vi "clipconf.vi"() -> ()   [LabVIEW 2009]
uses:
  <vilib>/Utility/NIReport.llb/NI_report.lvclass
  <instrlib>/Agilent 81150/Agilent 81150.lvlib
  <vilib>/Analysis/NI_AALBase.lvlib
panel:
  out "Instrument VISA out":T1
  in  "conf value":i32[](array[numeric])=[200, 220, 250, 180, 150, 120, 100, 300]
  in  "Fotoelecton to clip":i32[](array[numeric])=[0, 12, 11, 10, 9, 8, 7, 6]
  out "Numeric 3":i32
  out "error out":errorcluster
  out "Quantity bucle":i32=62
  out "mean value":dbl=711.9915188935893
  in  "Voltages comprobation":dbl[](array[numeric])=[0.05, 0.1, 0.2, 0.3, 0.35, 0.4, 0.45, 0.5, 0.55, 0.6, 0.7, 0.8, 0.9, 1.0, 1.2, 1.5, 1.8, 2.0]
  out "L1 values":i32[](array[numeric])=[75, 76, 78, 63, 67, 69]
  out "L1 values":i32[](array[numeric])=[350, 351, 357, 318, 319, 317]
  out "Vatt":i32[](array[numeric])=[2200, 2200, 2200, 2200, 2200, 2200]
  out "Vclip":i32[](array[numeric])=[415, 417, 409, 455, 424, 466]
  in  "Vatt ini":i32[](array[numeric])=[1500, 1500, 1500, 1500, 1500, 1500, 1500]
  in  "Vclip ini":i32[](array[numeric])=[0, 0, 0, 0, 0, 0, 0]
  in  "Comprobation":bool=TRUE
  in  "Channels":i32[](array[numeric])=[0, 1, 2, 3, 4, 5, 6]
  in  "Cycles Burst":i32=10000
  out "IPR_Address":i32=23
  out "L1 Address":i32=17
  in  "L1 version":bool
  in  "Instrument VISA in":T1={"AWG VISA"="81160A", "Oscilloscope  VISA "="DSO80204B", "Integration Board IP"="172.16.7.43", "connection ID"=refnum, "report out"=refnum, "report file path"=path "D:/CTA/Data_test"}
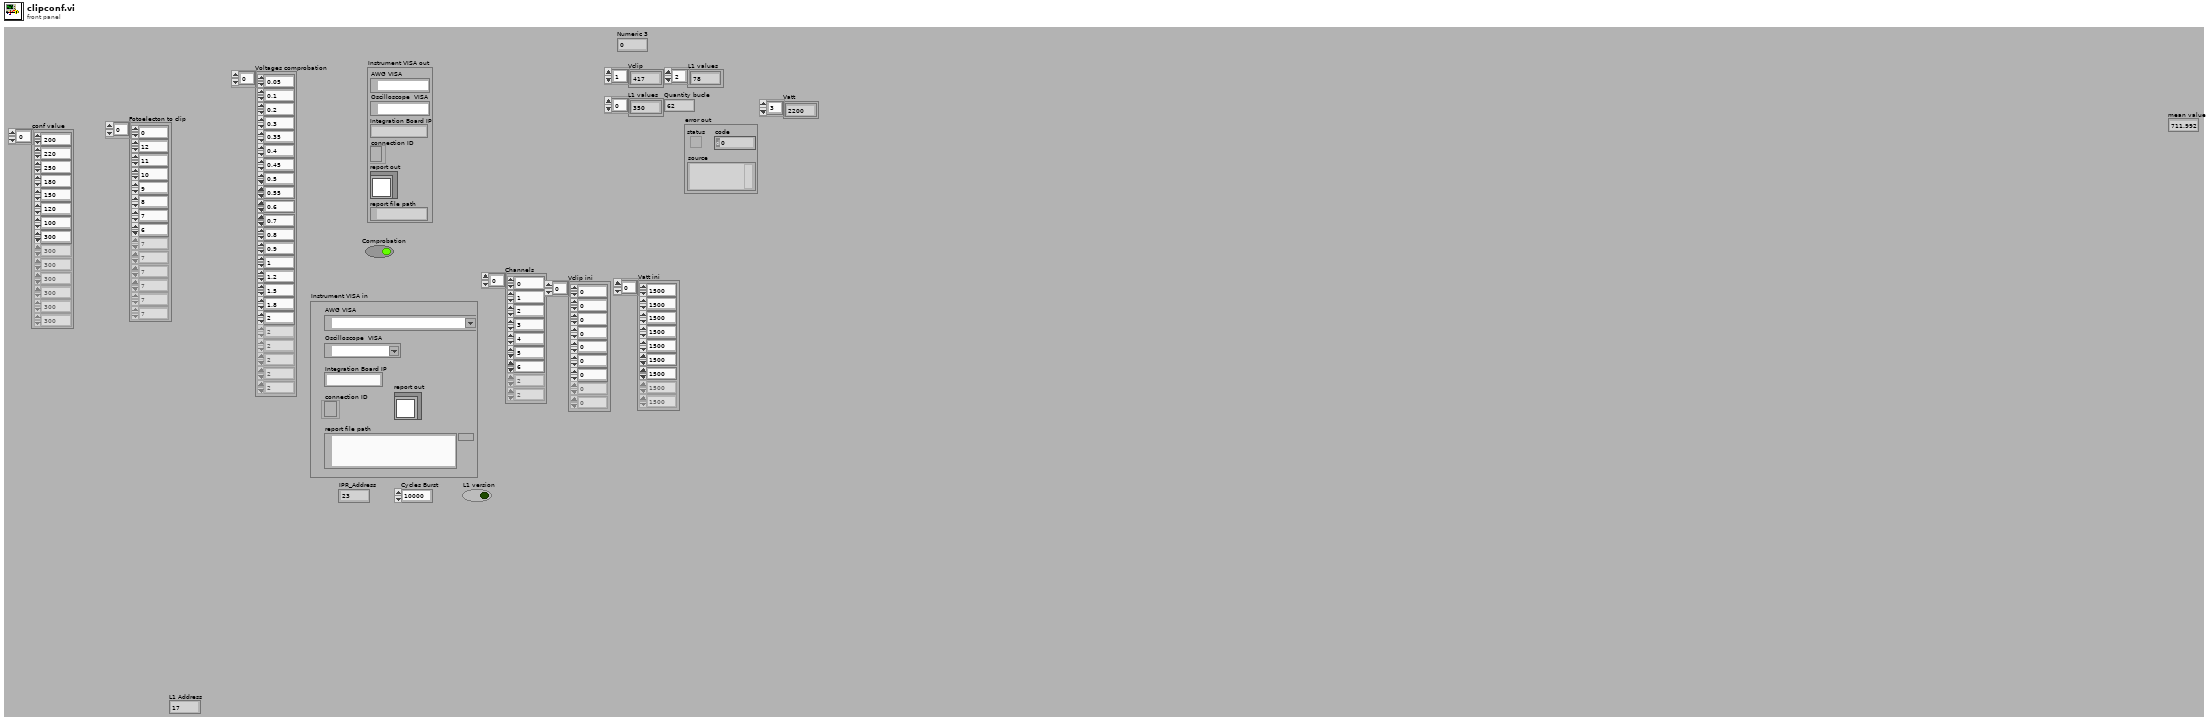
[diagram p1: front panel]
types:
  T1 = cluster{"AWG VISA":refnum<visa-resource-name>, "Oscilloscope  VISA ":refnum<visa-resource-name>, "Integration Board IP":string, "connection ID":refnum<k5>, "report out":refnum<class "NI_report.lvclass">, "report file path":path}
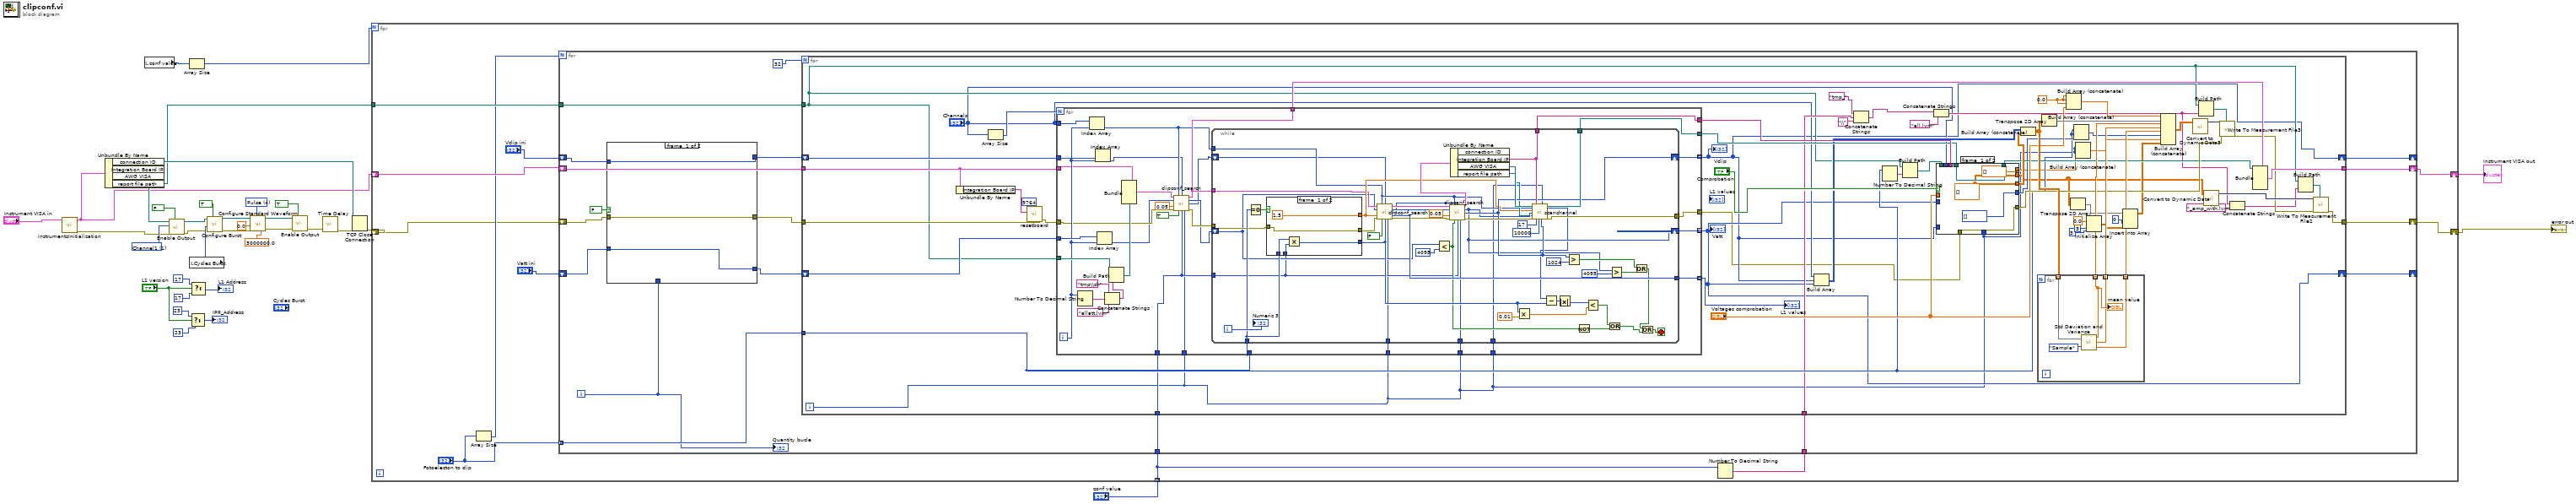
[diagram p0: block diagram]
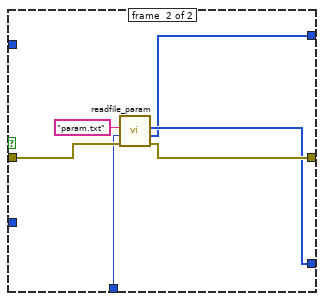
[diagram p2: hidden frame]
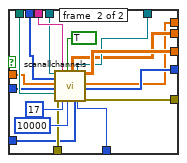
[diagram p3: hidden frame]
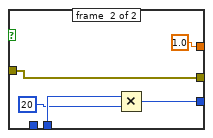
[diagram p4: hidden frame]
diagram:
  w26 = u16 4 items=["Sine", "Square", "Ramp Up", "Ramp Down", "Pulse", "Noise", "DC"] ("Waveform (0: Sine)")
  w32 = u16 1 items=["Channel1"=1, "Channel2"=2] ("Channel (1: Channel1)")
  n1 = call "instrumentsInitialization.vi"("Instrument VISA in"="Instrument VISA in") -> ("error out"=w11:errorcluster, "Instrument VISA out"=w1:T1)  [unwired: 9 in]
  n2 = Unbundle By Name(w1) -> ("connection ID"=w14:refnum<k5>, "AWG VISA"=w27:refnum<visa-resource-name>, "report file path"=w7:path)  [unwired: 1 out]
  n3 = local read "conf value"() -> (w35:i32[])
  n4 = call <instrlib>:"Enable Output.vi"("Enable Output (T: Enable)"=FALSE, "error in (no error)"=w11, "Channel (1: Channel1)"=w32, "VISA resource name"=w27) -> ("error out"=w13:errorcluster, "VISA resource name out"=w12:refnum<visa-resource-name>)  [unwired: 6 in]
  n5 = Array Size(array=w35) -> (size(s)=w5:i32)
  n6 = local read "Cycles Burst"() -> (w15:i32)
  n7 = Select(t=23 ("Address"), s="L1 version", f=23 ("Address")) -> (s? t:f=→"IPR_Address":i32)
  n8 = Select(t=17 ("Address"), s="L1 version", f=17 ("Address")) -> (s? t:f=→"L1 Address":i32)
  n9 = call <instrlib>:"Configure Burst.vi"("Enable Burst (F: Disable)"=TRUE, "error in (no error)"=w13, "Burst Count (2)"=w15, "VISA resource name"=w12) -> ("error out"=w23:errorcluster, "VISA resource name out"=w24:refnum<visa-resource-name>)  [unwired: 6 in]
  n10 = call <instrlib>:"Configure Standard Waveform.vi"("Frequency (1000.0 Hz)"=3000000.0, "Waveform (0: Sine)"=w26, "error in (no error)"=w23, "Amplitude (1.0 Vpp)"=0.0, "VISA resource name"=w24) -> ("error out"=w22:errorcluster, "VISA resource name out"=w10:refnum<visa-resource-name>)  [unwired: 5 in]
  n11 = call <instrlib>:"Enable Output.vi"("Enable Output (T: Enable)"=TRUE, "error in (no error)"=w22, "VISA resource name"=w10) -> ("error out"=w8:errorcluster)  [unwired: 7 in, 1 out]
  n12 = call "Time Delay"("error in (no error)"=w8) -> ("error out"=w9:errorcluster)  [unwired: 10 in]
  n13 = TCP Close Connection(connection ID=w14, error in (no error)=w9) -> (error out=w2:errorcluster)  [unwired: 1 in, 1 out]
  n14 = for {
    N: w5 -> [_]
    tunnel: w7 -> [w46]
    tunnel: "conf value" -> [w44] mode=indexing
    shift-right: [w43] -> w3
    shift-left: w1 -> [w42]
    shift-right: [w45] -> w6
    shift-left: w2 -> [w36]
    n15 = Array Size(array="Fotoelecton to clip") -> (size(s)=w40:i32)
    n16 = Number To Decimal String(number=w44) -> (decimal integer string=w39:string)  [unwired: 1 in]
    n17 = for {
      N: w40 -> [_]
      tunnel: w46 -> [w58]
      shift-right: [w56] -> _
      shift-left: "Vatt ini" -> [w52]
      shift-right: [w55] -> _
      shift-left: "Vclip ini" -> [w53]
      shift-right: [w64] -> w43
      shift-left: w42 -> [w63]
      shift-right: [w59] -> w45
      shift-left: w36 -> [w50]
      tunnel: "Fotoelecton to clip" -> [w62] mode=indexing
      tunnel: w44 -> [w61]
      tunnel: w39 -> [w60]
      i -> [w48]
      n18 = case shown="False" FALSE {
        tunnel: w50 -> [w67 w73]
        tunnel: [w67 w72] -> w49
        tunnel: [w65 w71] -> w51
        tunnel: [w66 w70] -> w54
        tunnel: w53 -> [w66 _]
        tunnel: w52 -> [w65 _]
        tunnel: w48 -> [_ w69]
        frame #0 {
        }
        frame #1 {
          n19 = call "readfile_param.vi"("error in"=w73, "index"=w69, "file"="param.txt") -> ("error out"=w72:errorcluster, "clipping"=w70:i32[], "attenuation"=w71:i32[])  [unwired: 4 in, 1 out]
        }
      }
      n20 = for {
        N: 32 -> [_]
        tunnel: [w123] -> w64
        tunnel: w49 -> [w111]
        tunnel: w63 -> [w109]
        tunnel: w62 -> [w103]
        tunnel: w61 -> [w102]
        tunnel: w60 -> [w98]
        tunnel: [w95] -> w59
        tunnel: w58 -> [w93]
        shift-right: [w77] -> w56
        shift-left: w51 -> [w135]
        shift-right: [w76] -> w55
        shift-left: w54 -> [w106]
        i -> [w75]
        w114 = 0.0 ("element")
        n21 = Unbundle By Name(w109) -> ("Integration Board IP"=w108:string)
        n22 = Array Size(array="Channels") -> (size(s)=w79:i32)
        n23 = call "resetboard.vi"("error in (no error)"=w111, "address"=w108, "remote port or service name"=u16 9764) -> ("error out"=w110:errorcluster)  [unwired: 7 in, 1 out]
        n24 = for {
          N: w79 -> [_]
          tunnel: w106 -> [w196]
          tunnel: "Channels" -> [w194]
          tunnel: w109 -> [w185]
          tunnel: w135 -> [w195]
          tunnel: [w189] -> w133
          tunnel: w93 -> [w198]
          tunnel: [w187] -> w77 mode=indexing
          tunnel: w110 -> [w178]
          tunnel: [w190] -> w74
          tunnel: [w183] -> w76 mode=indexing
          tunnel: [w188] -> w131 mode=indexing
          tunnel: [w182] -> w122
          tunnel: [w180] -> w124
          tunnel: w103 -> [w181]
          tunnel: w102 -> [w169]
          tunnel: w75 -> [w168]
          tunnel: w75 -> [w167]
          tunnel: w75 -> [w166]
          tunnel: w75 -> [w165]
          i -> [w186]
          n25 = Number To Decimal String(number=w186) -> (decimal integer string=w197:string)  [unwired: 1 in]
          n26 = Index Array(array=w194, index=w186) -> (element=w174:i32)
          n27 = Index Array(array=w196, index=w186) -> (element=w173:i32)
          n28 = Index Array(array=w195, index=w186) -> (element=w176:i32)
          n29 = Concatenate Strings("tmp\\ch" ("name or relative path"), w197, "allatt.lvm" ("string")) -> (w193:string)
          n30 = Build Path(base path=w198, name or relative path=w193) -> (appended path=w184:path)
          n31 = Bundle(cluster=w185, "report file path"=w184) -> (w179:T1)  [unwired: 5 in]
          n32 = call "clipconf_search.vi"("input cluster"=w179, "Channel"=w174, "vclip"=w173, "Vatt init"=w176, "Voltage value"=0.05, "error out 2"=w178, "Att/clip"=TRUE, "conf value"=w169, "Delay"=w168) -> ("output cluster"=w180:T1, "Vatt init"=w175:i32, "vclip"=w172:i32, "error out"=w177:errorcluster)  [unwired: 2 in, 1 out]
          n33 = while {
            tunnel: w177 -> [w208]
            tunnel: [w231] -> w190
            tunnel: [w234] -> w189
            tunnel: w174 -> [w206]
            shift-right: [w228] -> w183
            shift-left: w172 -> [w204]
            tunnel: [w247] -> w188
            shift-right: [w227] -> w187
            shift-left: w175 -> [w203]
            tunnel: w180 -> [w205]
            tunnel: [w233] -> w182
            tunnel: w181 -> [w212]
            tunnel: w169 -> [w202]
            tunnel: w167 -> [w201]
            tunnel: w166 -> [w200]
            tunnel: w165 -> [w199]
            i -> [w218]
            stop <- w246 stop-if-true
            n34 = Equal To 0?(x=w212) -> (x = 0?=w219:bool)
            n35 = case shown="False" w219 {
              tunnel: [1.5 ("Voltage value") 1.0 ("Voltage value")] -> w220
              tunnel: w202 -> [w250 w257]
              tunnel: [w251 w254] -> w213
              tunnel: w212 -> [w249 _]
              tunnel: w208 -> [w248 w253]
              tunnel: [w248 w253] -> w207
              frame #0 {
                n36 = Multiply(x=w249, y=w250) -> (x*y=w251:i32)
              }
              frame #1 {
                n37 = Multiply(x=w257, y=20) -> (x*y=w254:i32)
              }
            }
            n38 = call "clipconf_search.vi"("input cluster"=w205, "Channel"=w206, "vclip"=w204, "Vatt init"=w203, "Voltage value"=w220, "error out 2"=w207, "Att/clip"=FALSE, "conf value"=w213, "Delay"=w201) -> ("output cluster"=w241:T1, "Vatt init"=w239:i32, "vclip"=w211:i32, "L1 value"=w247:i32, "error out"=w242:errorcluster)  [unwired: 2 in]
            n39 = Less?(x=w203, y=4095) -> (x < y?=w210:bool)
            n40 = call "clipconf_search.vi"("input cluster"=w241, "Channel"=w206, "vclip"=w211, "Vatt init"=w239, "Voltage value"=0.05, "error out 2"=w242, "Att/clip"=w210, "conf value"=w202, "Delay"=w200) -> ("output cluster"=w240:T1, "Vatt init"=w227:i32, "vclip"=w228:i32, "error out"=w232:errorcluster)  [unwired: 2 in, 1 out]
            n41 = Unbundle By Name(w240) -> ("Integration Board IP"=w234:string, "AWG VISA"=w235:refnum<visa-resource-name>, "report file path"=w226:path)  [unwired: 1 out]
            n42 = Multiply(x=w213, y=0.01) -> (x*y=w221:dbl)
            n43 = call "scanchannel.vi"("VISA resource name out"=w235, "num ch"=w206, "Voltage value"=w220, "Init vatt value"=w227, "base path"=w226, "error in"=w232, "Integration Board IP"=w234, "L1 Address"=17, "Ch burst"=10000, "Delay"=w199, "vclip"=w228) -> ("VISA resource name out 2"=w233:refnum<visa-resource-name>, "L1 value"=w224:i32, "error out"=w231:errorcluster)  [unwired: 6 in]
            n44 = Subtract(x=w224, y=w213) -> (x-y=w225:i32)
            n45 = Absolute Value(x=w225) -> (abs(x)=w223:i32)
            n46 = Greater?(x=w228, y=1024) -> (0:w236:bool)
            n47 = Not(x=w210) -> (.not. x?=w214:bool)
            n48 = Less?(x=w223, y=w221) -> (x < y?=w216:bool)
            n49 = Or(x=w216, y=w214) -> (x .or. y?=w215:bool)
            n50 = Greater?(x=w227, y=4095) -> (0:w243:bool)
            n51 = Or(x=w236, y=w243) -> (x .or. y?=w245:bool)
            n52 = Or(x=w245, y=w215) -> (x .or. y?=w246:bool)
            "Numeric 3" <- w218
          }
        }
        "Vclip" <- w76
        "Vatt" <- w77
        "L1 values" <- w131
        n53 = Build Array("Channels", w76, w77) -> (w119:i32[][])
        n54 = Concatenate Strings("tmp_" ("name or relative path"), w98, "\\" ("name or relative path")) -> (w101:string)
        n55 = Number To Decimal String(number=w103) -> (decimal integer string=w125:string)  [unwired: 1 in]
        n56 = Build Path(base path=w93, name or relative path=w125) -> (appended path=w126:path)
        n57 = Concatenate Strings(w101, "all.lvm" ("string")) -> (w94:string)
        n58 = case shown="True" "Comprobation" {
          tunnel: [w146 w164] -> w117
          tunnel: w133 -> [_ w160]
          tunnel: w74 -> [w146 w159]
          tunnel: w126 -> [_ w158]
          tunnel: w76 -> [_ w157]
          tunnel: "Channels" -> [_ w156]
          tunnel: w77 -> [_ w155]
          tunnel: "Voltages comprobation" -> [_ w154]
          tunnel: [w143 w153] -> w120
          tunnel: w122 -> [w145 w152]
          tunnel: [w145 w151] -> w112
          tunnel: [u32[] [] ("time") w150] -> w104
          tunnel: [w143 w149] -> w81
          tunnel: [dbl[] [] ("temperatura") w148] -> w89
          tunnel: w75 -> [_ w147]
          frame #0 {
            w143 = dbl[][] [] ("L1  50%")
          }
          frame #1 {
            n59 = call "scanallchannels.vi"("VISA resource name in"=w152, "nm ch"=w156, "Voltages values"=w154, "Init ch value"=w155, "base path"=w158, "error in"=w159, "Integration Board IP"=w160, "L1 Address"=17, "Save test data"=TRUE, "Ch burst"=10000, "vclip"=w157, "Delay"=w147) -> ("Amp&width"=w149:dbl[][], "VISA resource name out"=w151:refnum<visa-resource-name>, "Array"=w153:dbl[][], "temperatura"=w148:dbl[], "time"=w150:u32[], "error out"=w164:errorcluster)  [unwired: 1 in, 1 out]
          }
        }
        n60 = Build Array (concatenate)(w119, w120) -> (w118:dbl[][])
        n61 = for {
          tunnel: w118 -> [w141] mode=indexing
          tunnel: [w139] -> w129 mode=indexing
          tunnel: [w138] -> w128 mode=indexing
          tunnel: [w137] -> w127 mode=indexing
          n62 = call <vilib>:"Std Deviation and Variance.vi"("X"=w141, "Weighting (Sample)"=enum16{"Sample", "Population"}."Sample") -> ("mean"=w139:dbl, "standard deviation"=w138:dbl, "variance"=w137:dbl)
          "mean value" <- w139
        }
        n63 = Transpose 2D Array(2D array=w118) -> (transposed array=w130:dbl[][])
        n64 = Build Array (concatenate)(w114, w114, w114, "Voltages comprobation") -> (w115:dbl[])
        n65 = Transpose 2D Array(2D array=w81) -> (transposed array=w87:dbl[][])
        n66 = Build Array (concatenate)(w103, w103, w103, w104) -> (w105:u32[])
        n67 = Build Array (concatenate)(w75, w75, w75, w89) -> (w88:dbl[])
        n68 = Initialize Array(0.0 ("element"), 3 ("dimension size"), 3 ("dimension size")) -> (w86:dbl[][])
        n69 = Insert Into Array(array=w87, index (col)=0 ("disabled index (col)"), new element=w86) -> (w82:dbl[][])  [unwired: 1 in]
        n70 = Build Array (concatenate)(w115, w130, w129, w128, w127, w105, w88, w82) -> (w121:dbl[][])
        n71 = call "Convert to Dynamic Data3"("2D Array"=w121) -> ("Dynamic Data Type"=w116:dynamicdata)  [unwired: 3 in]
        n72 = Build Path(base path=w93, name or relative path=w94) -> (appended path=w136:path)
        n73 = call "Convert to Dynamic Data"("2D Array"=w81) -> ("Dynamic Data Type"=w97:dynamicdata)  [unwired: 3 in]
        n74 = call "Write To Measurement File3"("Signals"=w116, "error in (no error)"=w117, "Filename"=w136) -> ("error out"=w96:errorcluster)  [unwired: 14 in, 2 out]
        n75 = Concatenate Strings(w94, "_amp_with.lvm" ("string")) -> (w91:string)
        n76 = Bundle(cluster=w124, "AWG VISA"=w112) -> (w123:T1)  [unwired: 5 in]
        n77 = Build Path(base path=w93, name or relative path=w91) -> (appended path=w90:path)
        n78 = call "Write To Measurement File2"("Signals"=w97, "error in (no error)"=w96, "Filename"=w90) -> ("error out"=w95:errorcluster)  [unwired: 14 in, 2 out]
      }
      "Quantity bucle" <- w48
    }
  }
  "error out" <- w6
  "Instrument VISA out" <- w3
